vi "Router - Latency Bmk - CVT.vi"() -> ()   [LabVIEW 2016]
uses:
  <vilib>/Utility/error.llb/DialogType.ctl
  <vilib>/NI/Current Value Table/Type Defs/File Format.ctl
  <vilib>/NI/Current Value Table/Type Defs/Single Tag.ctl
  <vilib>/NI/Current Value Table/Type Defs/Data Types.ctl
  <vilib>/NI/Current Value Table/Type Defs/Tag Grouping set.ctl
  <vilib>/NI/Current Value Table/DataTypes/Array of Double_Static Read.vi
  <vilib>/NI/Current Value Table/DataTypes/Array of Double_Static Write.vi
  <vilib>/NI/Current Value Table/Type to Enum.vi
  <vilib>/NI/Current Value Table/DataTypes/Array of Double_Type To Enum.vi
  <vilib>/pximc/Initialize Writer Session (DBL).vi
  <vilib>/pximc/Initialize Reader Session (DBL).vi
  <vilib>/pximc/Connect (DBL).vi
  <vilib>/NI/Current Value Table/FGVs/Tag Memory.vi
  <vilib>/NI/Current Value Table/Memory Block.vi
  <vilib>/NI/Current Value Table/DataTypes/Array of Double_Memory Block.vi
  <vilib>/pximc/Write (DBL).vi
  <vilib>/pximc/Read (DBL).vi
  <vilib>/pximc/nipximc.lvlib
  <vilib>/NI/Current Value Table/Current Value Table.lvlib
panel:
  out "Stopped?":bool
  in  "Node 2 Reader Interface":tag="PXI1Slot2" caption="interface"
  in  "Node 2 Reader Connection ID":u16=4
  in  "Node 2 Writer Interface":tag="PXI1Slot2" caption="interface"
  in  "Node 2 Writer Connection ID":u16=3
  in  "Node 1 Reader Interface":tag="PXI1Slot2" caption="interface"
  in  "Node 1 Reader Connection ID":u16=2
  in  "Stop Button":bool
  in  "Node 1 Writer Interface":tag="PXI1Slot2" caption="interface"
  in  "Buffer Size":u64=250000 caption="buffer size"
  in  "Connection Timeout (s)":dbl=60.0 caption="timeout in seconds (-1)"
  in  "Node 1 Writer Connection ID":u16=1
  # "Node 1"
  # "Node 2"
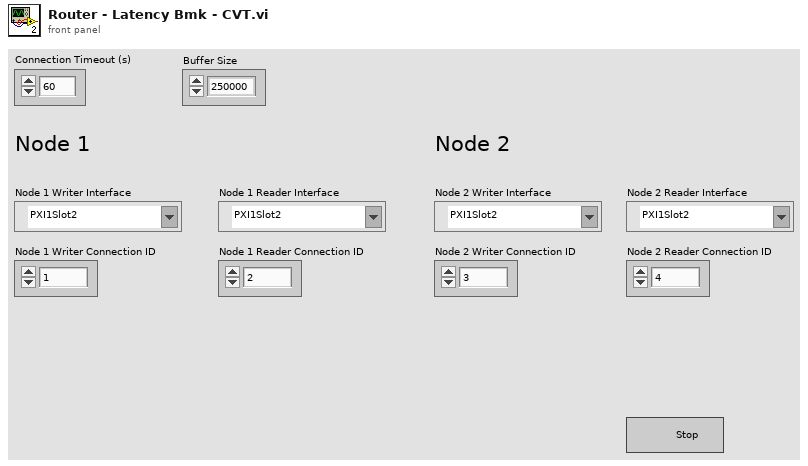
[diagram p1: front panel]
types:
  T1 = typedef "Current Value Table.lvlib/File Format.ctl" = cluster{"Tags":T2[], "Group Listings":T4[]}
  T2 = typedef "Current Value Table.lvlib/Single Tag.ctl" = cluster{"Data Type":T3, "Name":string, "Value":string, "Description":string}
  T3 = typedef "Current Value Table.lvlib/Data Types.ctl" = enum16{"Double", "Single", "I64", "I32", "I16", "I8", "U64", "U32", "U16", "U8", "String", "Boolean", "Array of U8", "Array of U16", "Array of U32", "Array of U64", "Array of I64", "Array of I32", "Array of I16", "Array of I8", "Array of Double", "Array of Single", "Array of Boolean", "Array of String"}
  T4 = typedef "Current Value Table.lvlib/Tag Grouping set.ctl" = cluster{"Group":string, "Tag Names":string[]}
  T5 = typedef "DialogType.ctl" = u16
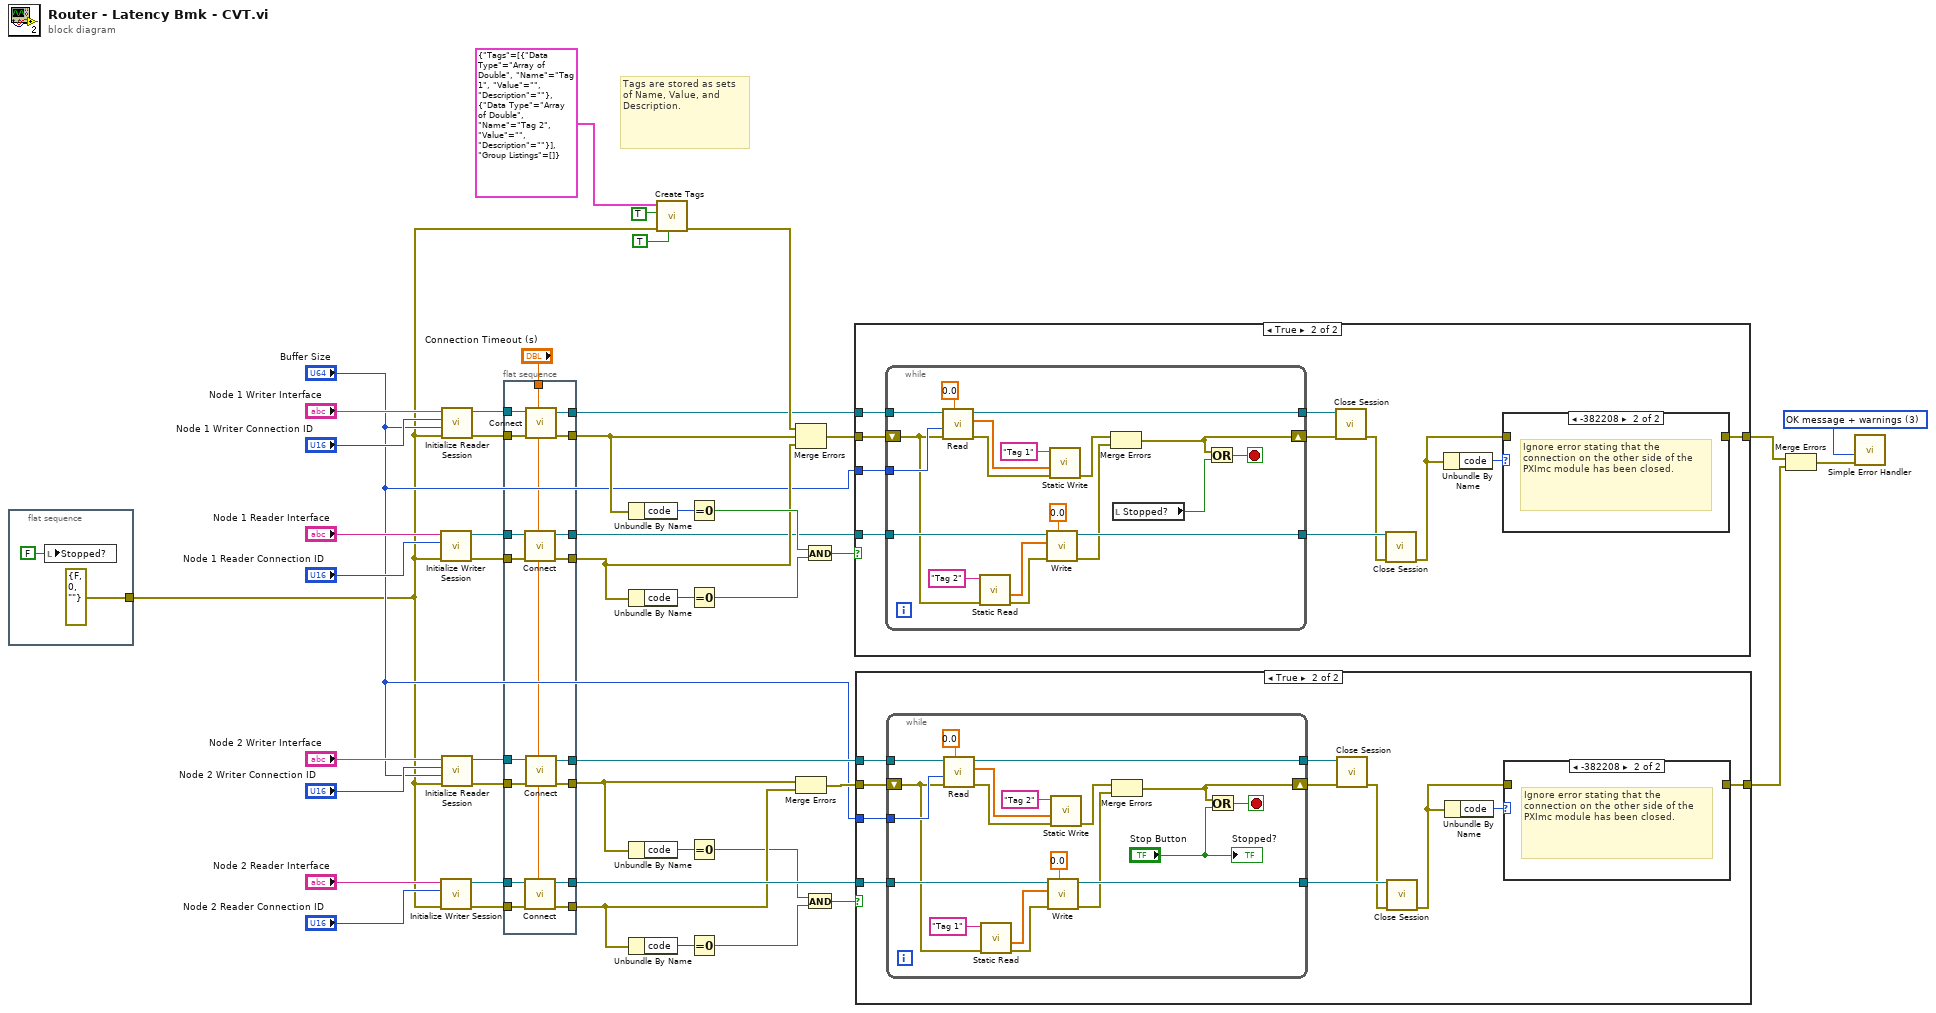
[diagram p0: block diagram]
diagram:
  w42 = T5 3 items=["no dialog", "OK message", "continue or stop message", "OK message + warnings", "continue/stop + warnings"] ("type of dialog (OK msg:1)")
  # "Tags are stored as sets of Name, Value, and Description."
  n1 = flat-sequence {
    tunnel: [errorcluster {"status"=FALSE, "code"=0, "source"=""} ("error constant")] -> w1
    frame #0 {
      n2 = local write "Stopped?"(FALSE ("Stopped?")) -> ()
    }
  }
  n3 = call-poly <vilib>:"Initialize Writer Session.vi"("error in (no error)"=w1, "connection id (1)"="Node 1 Reader Connection ID", "interface"="Node 1 Reader Interface") -> ("error out"=w40:errorcluster, "session out"=w39:refnum<k21>)  [unwired: 7 in]
  n4 = call-poly <vilib>:"Initialize Writer Session.vi"("error in (no error)"=w1, "connection id (1)"="Node 2 Reader Connection ID", "interface"="Node 2 Reader Interface") -> ("error out"=w21:errorcluster, "session out"=w22:refnum<k21>)  [unwired: 7 in]
  n5 = call-poly <vilib>:"Initialize Reader Session.vi"("error in (no error)"=w1, "buffer size"="Buffer Size", "writer's connection id (1)"="Node 1 Writer Connection ID", "interface"="Node 1 Writer Interface") -> ("error out"=w45:errorcluster, "session out"=w46:refnum<k21>)  [unwired: 6 in]
  n6 = call-poly <vilib>:"Initialize Reader Session.vi"("error in (no error)"=w1, "buffer size"="Buffer Size", "writer's connection id (1)"="Node 2 Writer Connection ID", "interface"="Node 2 Writer Interface") -> ("error out"=w16:errorcluster, "session out"=w15:refnum<k21>)  [unwired: 6 in]
  n7 = flat-sequence {
    tunnel: w46 -> [w66]
    tunnel: w45 -> [w65]
    tunnel: [w64] -> w7
    tunnel: w40 -> [w63]
    tunnel: w39 -> [w62]
    tunnel: [w61] -> w34
    tunnel: [w60] -> w33
    tunnel: "Connection Timeout (s)" -> [w50]
    tunnel: [w59] -> w4
    tunnel: [w58] -> w31
    tunnel: [w57] -> w30
    tunnel: [w56] -> w29
    tunnel: w22 -> [w55]
    tunnel: w21 -> [w54]
    tunnel: [w53] -> w17
    tunnel: w16 -> [w52]
    tunnel: w15 -> [w51]
    frame #0 {
      n8 = call-poly <vilib>:"Connect.vi"("timeout in seconds (-1)"=w50, "error in (no error)"=w63, "session in"=w62) -> ("error out"=w60:errorcluster, "session out"=w59:refnum<k21>)  [unwired: 7 in]
      n9 = call-poly <vilib>:"Connect.vi"("timeout in seconds (-1)"=w50, "error in (no error)"=w54, "session in"=w55) -> ("error out"=w57:errorcluster, "session out"=w58:refnum<k21>)  [unwired: 7 in]
      n10 = call-poly <vilib>:"Connect.vi"("timeout in seconds (-1)"=w50, "error in (no error)"=w65, "session in"=w66) -> ("error out"=w61:errorcluster, "session out"=w64:refnum<k21>)  [unwired: 7 in]
      n11 = call-poly <vilib>:"Connect.vi"("timeout in seconds (-1)"=w50, "error in (no error)"=w52, "session in"=w51) -> ("error out"=w56:errorcluster, "session out"=w53:refnum<k21>)  [unwired: 7 in]
    }
  }
  n12 = Unbundle By Name(w34) -> ("code"=w43:i32)
  n13 = Unbundle By Name(w33) -> ("code"=w37:i32)
  n14 = Unbundle By Name(w29) -> ("code"=w19:i32)
  n15 = Unbundle By Name(w30) -> ("code"=w24:i32)
  n16 = call <vilib>:"Create Tags.vi"("Overwrite Duplicates? (F)"=TRUE, "error in (no error)"=w1, "Clear Table? (F)"=TRUE ("Clear Engine?"), "CVT Tags to Create"=T1 {"Tags"=[{"Data Type"=enum."Array of Double", "Name"="Tag 1", "Value"="", "Description"=""}, {"Data Type"=enum."Array of Double", "Name"="Tag 2", "Value"="", "Description"=""}], "Group Listings"=[]} ("CVT File Data")) -> ("error out"=w9:errorcluster)  [unwired: 7 in]
  n17 = Equal To 0?(x=w43) -> (x = 0?=w36:bool)
  n18 = Equal To 0?(x=w37) -> (x = 0?=w35:bool)
  n19 = Equal To 0?(x=w19) -> (x = 0?=w26:bool)
  n20 = Equal To 0?(x=w24) -> (x = 0?=w27:bool)
  n21 = Merge Errors(w9, w34, w33) -> (w6:errorcluster)
  n22 = Merge Errors(w29, w30) -> (w28:errorcluster)
  n23 = And(x=w36, y=w35) -> (x .and. y?=w3:bool)
  n24 = And(x=w26, y=w27) -> (x .and. y?=w25:bool)
  n25 = case shown="True" w3 {
    tunnel: w6 -> [w67 w78]
    tunnel: w7 -> [_ w77]
    tunnel: [w67 w75] -> w8
    tunnel: w4 -> [_ w72]
    tunnel: "Buffer Size" -> [_ w68]
    frame False {
      # "The connection was not successful for some reason."
    }
    frame True {
      n26 = while {
        tunnel: w77 -> [w97]
        tunnel: [w96] -> w76
        shift-right: [w91] -> w73
        shift-left: w78 -> [w83]
        tunnel: w72 -> [w95]
        tunnel: [w94] -> w71
        tunnel: w68 -> [w88]
        stop <- w92 stop-if-true
        n27 = call-poly <vilib>:"Read.vi"("timeout in seconds (5)"=0.0, "error in (no error)"=w83, "number of elements"=w88, "session in"=w97) -> ("error out"=w85:errorcluster, "data"=w87:dbl[], "session out"=w96:refnum<k21>)  [unwired: 5 in]
        n28 = call-poly <vilib>:"Static Read.vi"("error in (no error)"=w83, "Tag Name"="Tag 2") -> ("error out"=w81:errorcluster, "Value"=w80:dbl[])  [unwired: 8 in]
        n29 = call-poly <vilib>:"Write.vi"("timeout in seconds (5)"=0.0, "error in (no error)"=w81, "data"=w80, "session in"=w95) -> ("error out"=w93:errorcluster, "session out"=w94:refnum<k21>)  [unwired: 5 in, 1 out]
        n30 = call-poly <vilib>:"Static Write.vi"("error in (no error)"=w85, "Value"=w87, "Tag Name"="Tag 1") -> ("error out"=w84:errorcluster)  [unwired: 8 in]
        n31 = Merge Errors(w84, w93) -> (w91:errorcluster)
        n32 = local read "Stopped?"() -> (w79:bool)
        n33 = Or(x=w91, y=w79) -> (x .or. y?=w92:bool)
      }
      n34 = call <vilib>:"Close Session.vi"("error in (no error)"=w73, "session in"=w76) -> ("error out"=w70:errorcluster)  [unwired: 9 in]
      n35 = call <vilib>:"Close Session.vi"("error in (no error)"=w70, "session in"=w71) -> ("error out"=w69:errorcluster)  [unwired: 9 in]
      n36 = Unbundle By Name(w69) -> ("code"=w74:i32)
      n37 = case shown="-382208" w74 {
        tunnel: w69 -> [w98 _]
        tunnel: [w98 _] -> w75
        frame 0, Default {
        }
        frame -382208 {
          # "Ignore error stating that the connection on the other side of the PXImc module has been closed."
        }
      }
    }
  }
  n38 = case shown="True" w25 {
    tunnel: w28 -> [w99 w110]
    tunnel: w17 -> [_ w109]
    tunnel: [w99 w107] -> w13
    tunnel: w31 -> [_ w104]
    tunnel: "Buffer Size" -> [_ w100]
    frame False {
      # "The connection was not successful for some reason."
    }
    frame True {
      n39 = while {
        tunnel: w109 -> [w129]
        tunnel: [w128] -> w108
        shift-right: [w123] -> w105
        shift-left: w110 -> [w115]
        tunnel: w104 -> [w127]
        tunnel: [w126] -> w103
        tunnel: w100 -> [w120]
        stop <- w124 stop-if-true
        n40 = call-poly <vilib>:"Read.vi"("timeout in seconds (5)"=0.0, "error in (no error)"=w115, "number of elements"=w120, "session in"=w129) -> ("error out"=w117:errorcluster, "data"=w119:dbl[], "session out"=w128:refnum<k21>)  [unwired: 5 in]
        n41 = call-poly <vilib>:"Static Read.vi"("error in (no error)"=w115, "Tag Name"="Tag 1") -> ("error out"=w113:errorcluster, "Value"=w112:dbl[])  [unwired: 8 in]
        n42 = call-poly <vilib>:"Write.vi"("timeout in seconds (5)"=0.0, "error in (no error)"=w113, "data"=w112, "session in"=w127) -> ("error out"=w125:errorcluster, "session out"=w126:refnum<k21>)  [unwired: 5 in, 1 out]
        n43 = call-poly <vilib>:"Static Write.vi"("error in (no error)"=w117, "Value"=w119, "Tag Name"="Tag 2") -> ("error out"=w116:errorcluster)  [unwired: 8 in]
        n44 = Merge Errors(w116, w125) -> (w123:errorcluster)
        n45 = Or(x=w123, y="Stop Button") -> (x .or. y?=w124:bool)
        "Stopped?" <- "Stop Button"
      }
      n46 = call <vilib>:"Close Session.vi"("error in (no error)"=w105, "session in"=w108) -> ("error out"=w102:errorcluster)  [unwired: 9 in]
      n47 = call <vilib>:"Close Session.vi"("error in (no error)"=w102, "session in"=w103) -> ("error out"=w101:errorcluster)  [unwired: 9 in]
      n48 = Unbundle By Name(w101) -> ("code"=w106:i32)
      n49 = case shown="-382208" w106 {
        tunnel: w101 -> [w130 _]
        tunnel: [w130 _] -> w107
        frame 0, Default {
        }
        frame -382208 {
          # "Ignore error stating that the connection on the other side of the PXImc module has been closed."
        }
      }
    }
  }
  n50 = Merge Errors(w8, w13) -> (w12:errorcluster)
  n51 = call <vilib>:"Simple Error Handler.vi"("type of dialog (OK msg:1)"=w42, "error in (no error)"=w12) -> ()  [unwired: 3 in, 5 out]
